vi "H5Dcreate.vi"(0 "file_id":i32, 3 "error in (no error)":errorcluster, 4 "space_id":i32, 6 "name":string) -> (7 "dset_id":i32, 10 "error out":errorcluster)   [LabVIEW 2009]
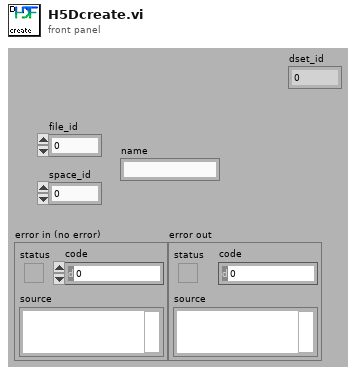
[diagram p1: front panel]
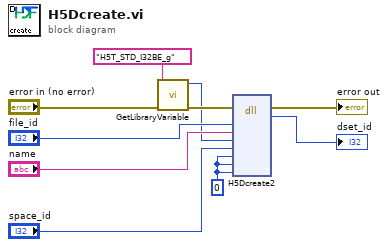
[diagram p0: block diagram]
diagram:
  w6 = 0 ("lcpl_id")
  n1 = call "GetLibraryVariable.vi"("Parameter"="H5T_STD_I32BE_g", "error in (no error)"="error in (no error)") -> ("Value"=w2:i32, "error out"=w4:errorcluster)  [unwired: 6 in]
  n2 = dll-call lib="hdf5dll" fn="H5Dcreate2"(error in=w4, "loc_id"="file_id", "name"="name", "type_id"=w2, "space_id"="space_id", "lcpl_id"=w6, "dcpl_id"=w6, "dapl_id"=w6) -> (error out=→"error out":errorcluster, "return type"=→"dset_id":i32)  [unwired: 9 in, 1 out]
